vi "Shoot Fuel.vi"   [LabVIEW 2025]
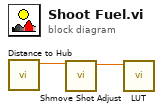
[diagram p0: block diagram]
diagram:
  n1 = call "Distance to Hub.vi"() -> ("Distance to Hub (ft)"=w2:dbl)  [unwired: 10 in, 1 out]
  n2 = call "Shmove Shot Adjust.vi"("Hub Distance"=w2) -> ("Adjusted Hub Distance"=w1:dbl)  [unwired: 10 in]
  n3 = call "LUT.vi"("Hub Distance (ft)"=w1) -> ()  [unwired: 9 in, 2 out]
